vi "target.vi"() -> ()   [LabVIEW 2020]
uses:
  <vilib>/rvi/interface/RandomDataEmulation/niFpgaRandomDataHandleErrors.vi
  <vilib>/rvi/DataTransferAndStorage/Container/XNode/niFpgaContainer.xnode
  <vilib>/rvi/interface/RandomDataEmulation/nirviRandomDataFpgaReadWriteTemplate.vi
panel:
  out "Timed Out? FIFO in REAL":bool
  out "Timed Out? FIFO out REAL":bool
  out "sort time (us)":u32
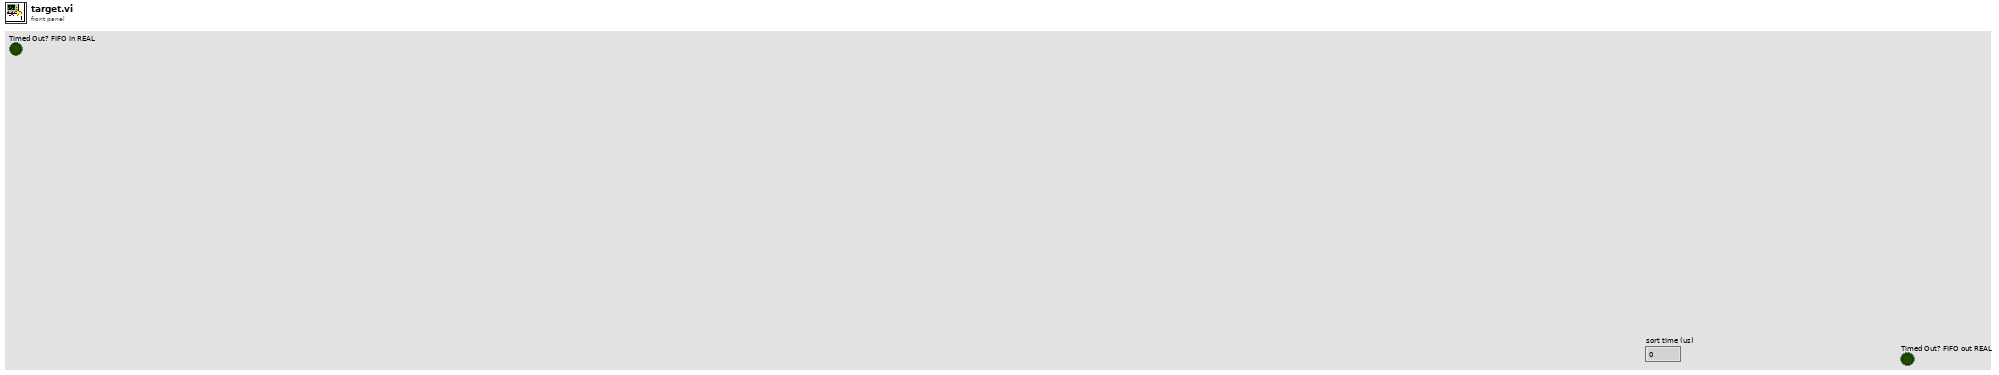
[diagram p1: front panel]
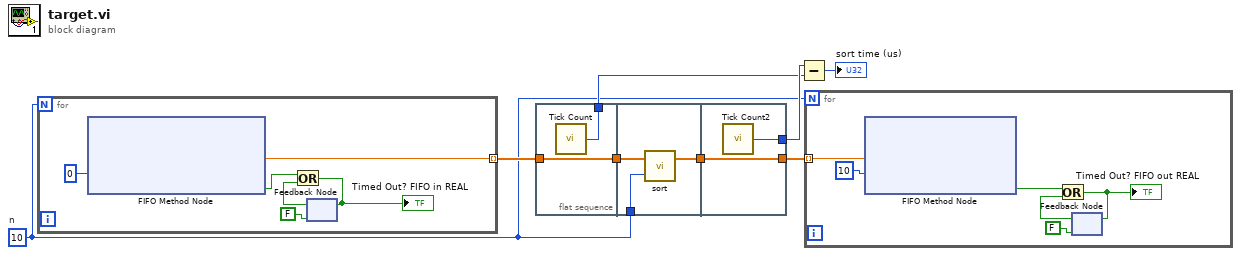
[diagram p0: block diagram]
diagram:
  w1 = 10  # n
  n1 = for {
    N: w1 -> [_]
    tunnel: [w9] -> w5 mode=indexing
    n2 = xnode ("FIFO Method Node")("Timeout"=0) -> ("Element"=w9:sgl, "Timed Out?"=w10:bool)  [unwired: 1 in, 1 out]
    n3 = feedback #1(FALSE) -> (w11:bool)
    n4 = Or(x=w10, y=w11) -> (x .or. y?=w12:bool)
    "Timed Out? FIFO in REAL" <- w12
    n5 = feedback-in #1(w12) -> ()
  }
  n6 = flat-sequence {
    tunnel: [w16] -> w7
    tunnel: w5 -> [w15]
    tunnel: [w15] -> w4
    tunnel: w1 -> [w19]
    tunnel: w4 -> [w17]
    tunnel: [w18] -> w3
    tunnel: [w21] -> w8
    tunnel: [w20] -> w2
    tunnel: w3 -> [w20]
    frame #0 {
      n7 = call "Tick Count"() -> ("Tick Count(uSec)"=w16:u32)
    }
    frame #1 {
      n8 = call "sort.vi"("n"=w19, "Real"=w17) -> ("Sorted A"=w18:sgl[])  [unwired: 1 in]
    }
    frame #2 {
      n9 = call "Tick Count2"() -> ("Tick Count(uSec)"=w21:u32)
    }
  }
  n10 = Subtract(x=w8, y=w7) -> (x-y=→"sort time (us)":u32)
  n11 = for {
    N: w1 -> [_]
    tunnel: w2 -> [w27] mode=indexing
    n12 = xnode ("FIFO Method Node")("Element"=w27, "Timeout"=10) -> ("Timed Out?"=w22:bool)  [unwired: 1 in, 1 out]
    n13 = feedback #2(FALSE) -> (w23:bool)
    n14 = Or(x=w22, y=w23) -> (x .or. y?=w24:bool)
    "Timed Out? FIFO out REAL" <- w24
    n15 = feedback-in #2(w24) -> ()
  }
